vi "Send_Msj_Nplot.vi"(4 "ItemNames":string[][](array[string]), 5 "Process in":i32, 6 "Send message":bool, 7 "msj":string, 8 "error in (no error)":errorcluster, 9 "queue in":refnum<queue>) -> (0 "error out":errorcluster)   [LabVIEW 2022 SP3]
panel:
  # "temporal function to send message to each process"
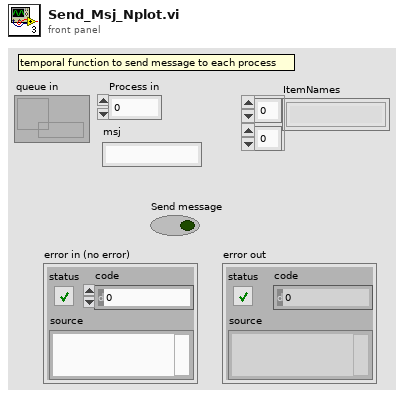
[diagram p1: front panel]
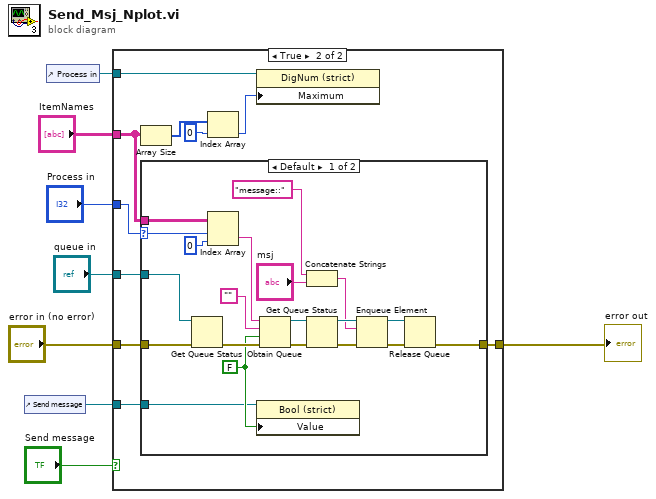
[diagram p0: block diagram]
diagram:
  n1 = control-ref of="Send message"() -> (w3:refnum<vi>)
  n2 = control-ref of="Process in"() -> (w2:refnum<vi>)
  n3 = case shown="True" "Send message" {
    tunnel: "ItemNames" -> [_ w17]
    tunnel: "error in (no error)" -> [w9 w19]
    tunnel: "queue in" -> [_ w18]
    tunnel: "Process in" -> [_ w13]
    tunnel: w3 -> [_ w12]
    tunnel: w2 -> [_ w11]
    tunnel: [w9 w10] -> w1
    frame False {
    }
    frame True {
      n4 = Array Size(array=w17) -> (size(s)=w15:i32[])
      n5 = case shown="Default" w13 {
        selector: w13 -> [w37 _]
        tunnel: w17 -> [w39 _]
        tunnel: w19 -> [w28 w40]
        tunnel: w18 -> [w29 _]
        tunnel: w12 -> [w21 _]
        tunnel: [w20 w40] -> w10
        frame Default {
          w24 = FALSE ("create if not found? (T)")
          n6 = Get Queue Status(queue=w29, error in (no error)=w28) -> (error out=w26:errorcluster)  [unwired: 1 in, 7 out]
          n7 = Index Array(array=w39, index (row)=w37, index (col)=0 ("disabled index (col)")) -> (element=w22:string)
          n8 = property class="Bool (strict)"(reference=w21, "Value"=w24) -> ()  [unwired: 1 in, 2 out]
          n9 = Obtain Queue(name (unnamed)=w22, element data type="", create if not found? (T)=w24, error in (no error)=w26) -> (queue out=w27:refnum<queue>, error out=w25:errorcluster)  [unwired: 1 in, 1 out]
          n10 = Concatenate Strings("message::", "msj") -> (w32:string)
          n11 = Get Queue Status(queue=w27, error in (no error)=w25) -> (queue out=w36:refnum<queue>, error out=w35:errorcluster)  [unwired: 1 in, 6 out]
          n12 = Enqueue Element(queue=w36, element=w32, error in (no error)=w35) -> (queue out=w31:refnum<queue>, error out=w30:errorcluster)  [unwired: 1 in, 1 out]
          n13 = Release Queue(queue=w31, error in (no error)=w30) -> (error out=w20:errorcluster)  [unwired: 1 in, 2 out]
        }
        frame ..-1 {
        }
      }
      n14 = Index Array(array=w15, index=0) -> (element=w14:i32)
      n15 = property on="Property Node" class="DigNum (strict)"(reference=w11, "Maximum"=w14) -> ()  [unwired: 1 in, 2 out]
    }
  }
  "error out" <- w1
